vi "P2P SPI Slave.vi"   [LabVIEW 2015]
uses:
  <vilib>/Platform/TimedLoop/XDataNode/timing_clust.ctl
  <vilib>/Platform/TimedLoop/XDataNode/nitl_modes.ctl
  <vilib>/Platform/TimedLoop/XDataNode/wakeup.ctl
  <vilib>/rvi/Emulation/niFpgaSctlEmulationGetInTimedLoop.vi
  <vilib>/rvi/Emulation/niFpgaEmulationReportErrorSimple.vi
  <vilib>/rvi/Emulation/niFpgaGetClockAttributes.vi
  <vilib>/rvi/Emulation/niFpgaCriticalErrorInLSC.vi
  <vilib>/rvi/eio/common/nirviEmuTemplateMethod_errors.vi
  <vilib>/rvi/Emulation/niFpgaEmulationIsFPGAContextNoSignature.vi
  <vilib>/rvi/errors/niFpgaSetErrorForExecOnDevCompSimple.vi
  <vilib>/rvi/eio/common/nirviEmuReportErrorAndStop.vi
  <vilib>/rvi/DataTransferAndStorage/Container/Common/niFpgaContainerGetUniqueNameForEmu.vi
  <vilib>/rvi/FIFO/Fifo_Resource/nirvififoEmulationSetSize.vi
  <vilib>/rvi/FIFO/Fifo_Resource/nirviFifoEmulationQueueMgr.vi
  <instcachedir>/0/nirviFifoEmulationQueueMgr_E5CAEC123FF24DC58D834DCA3CDAA9B5.lvgen/nirviFifoEmulationQueueMgr_E5CAEC123FF24DC58D834DCA3CDAA9B5_001.vi
  <vilib>/rvi/FIFO/Fifo_Resource/nirvififoEmulationDetermineInputValidOut.vi
  <vilib>/rvi/FIFO/Fifo_Resource/nirvififoEmulationCreateLock.vi
  <vilib>/rvi/Emulation/niFpgaProcessEmulError.vi
  <vilib>/rvi/FIFO/Fifo_Resource/nirvififoEmulationObtainLock.vi
  <vilib>/rvi/FIFO/Fifo_Resource/nirvififoEmulationReleaseLock.vi
  <vilib>/rvi/occurrence/nirviWaitOnOccurrenceBase.vi
  <vilib>/rvi/errors/nirviReportUnexpectedCaseInternalError.vi
  <vilib>/rvi/errors/nirviReportUnexpectedCaseInternalError (U32).vi
  <vilib>/Platform/TimedLoop/XDataNode/XDataNode.xnode
  <vilib>/eio/EIONode/EIONode.xnode
  <vilib>/rvi/DataTransferAndStorage/Container/XNode/niFpgaContainer.xnode
  <vilib>/rvi/FIFO/Fifo_Resource/nirvififoEmulationWrite.vi
  <vilib>/Platform/TimedLoop/XDataNode/XDNodeRunTimeDep.lvlib
types:
  T1 = typedef "XDNodeRunTimeDep.lvlib/timing_clust.ctl" = cluster{"Expected End [f-1]":u64, "Actual End [f-1]":u64, "Finished Late? [f-1]":bool, "Expected End [i-1]":u64, "Actual End [i-1]":u64, "Finished Late? [i-1]":bool, "Expected Start [i]":u64, "Actual Start [i]":u64, "Expected Start [f]":u64, "Actual Start [f]":u64, "Source Name":string, "Structure Name":string, "Period":i64, "Deadline":i64, "Offset":i64, "Start":i64, "Priority":i32, "Timeout":i32, "Mode":T2, "Wakeup Reason":T3, "Error":errorcluster, "Source Type":string, "Secondary Source Type":string, "Global End Time":u64, "Global Start Time":u64, "Frame Duration":u64, "Iteration Duration":u64, "Assigned CPU":i32, "I/O Scan Engine Mode":u32}
  T2 = typedef "XDNodeRunTimeDep.lvlib/nitl_modes.ctl" = enum32{"No Change", "Process missed periods, maintain original phase", "Discard missed periods, maintain original phase", "Process missed periods, ignore original phase", "Discard missed periods, ignore original phase"}
  T3 = typedef "XDNodeRunTimeDep.lvlib/wakeup.ctl" = enum32{"Normal", "Aborted", "Asynchronous wakeup", "Timing source error", "Timed loop error", "Timeout"}
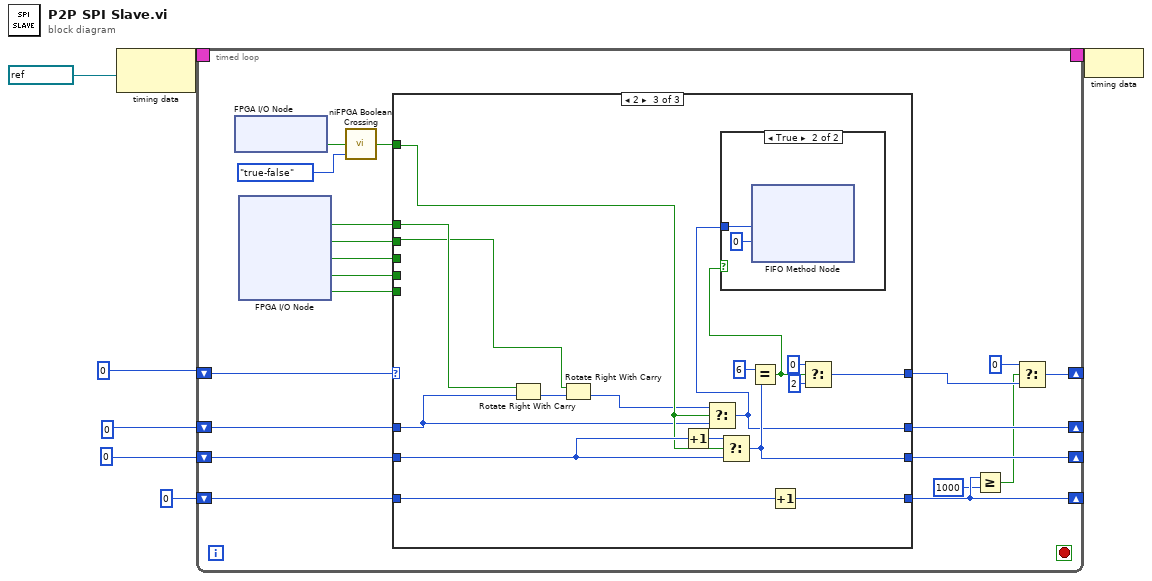
[diagram p0: block diagram]
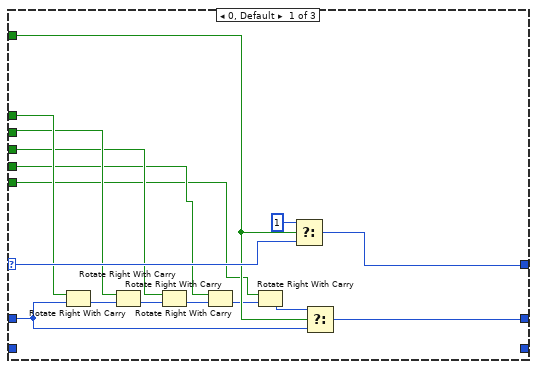
[diagram p2: hidden frame]
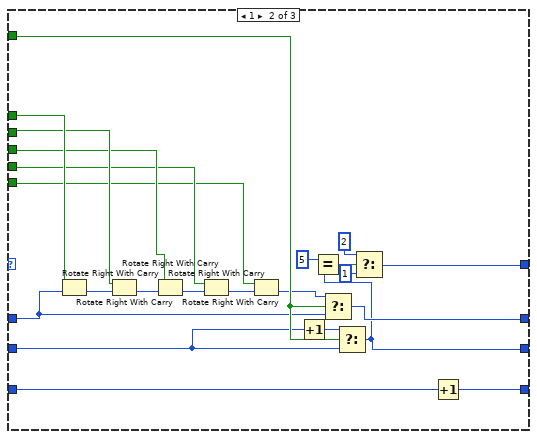
[diagram p3: hidden frame]
diagram:
  n1 = node-c288(refnum<k21> "80MHz" ("Source Name")) -> (w7:T1)
  n2 = timed-loop {
    timing: w7 -> [_]
    timing-out: [_] -> w6
    shift-right: [w9] -> _
    shift-left: u8 0 -> [w27]
    shift-right: [w21] -> _
    shift-left: u32 0 -> [w23]
    shift-right: [w11] -> _
    shift-left: u8 0 -> [w20]
    shift-right: [w14] -> _
    shift-left: 0 -> [w15]
    stop <- _ stop-if-true
    n3 = xnode "FPGA I/O Node"() -> ("PXI_Trig2"=w26:bool)  [unwired: 1 in, 1 out]
    n4 = xnode "FPGA I/O Node"() -> ("PXI_Trig3"=w22:bool, "PXI_Trig4"=w19:bool, "PXI_Trig5"=w18:bool, "PXI_Trig6"=w17:bool, "PXI_Trig7"=w16:bool)  [unwired: 5 in, 5 out]
    n5 = call <vilib>:"niFPGA Boolean Crossing.vi"("input"=w26, "direction"=enum8{"either", "false-true", "true-false"}."true-false") -> ("crossing"=w25:bool)  [unwired: 7 in]
    n6 = case shown="2" w27 {
      selector: w27 -> [w42 _ _]
      tunnel: w25 -> [w40 w65 w76]
      tunnel: [w43 w62 w81] -> w10
      tunnel: w23 -> [w33 w49 w70]
      tunnel: w22 -> [w32 w48 w69]
      tunnel: [w39 w64 w74] -> w21
      tunnel: w20 -> [_ w61 w80]
      tunnel: [_ w60 w79] -> w11
      tunnel: w19 -> [w31 w47 w68]
      tunnel: w18 -> [w30 w46 _]
      tunnel: w17 -> [w29 w45 _]
      tunnel: w16 -> [w28 w44 _]
      tunnel: [_ w55 w72] -> w14
      tunnel: w15 -> [_ w56 w73]
      frame 0, Default {
        n7 = Rotate Right With Carry(2:w33, 3:w32) -> (0:w35:u32)  [unwired: 1 out]
        n8 = Rotate Right With Carry(2:w35, 3:w31) -> (0:w36:u32)  [unwired: 1 out]
        n9 = Rotate Right With Carry(2:w36, 3:w30) -> (0:w37:u32)  [unwired: 1 out]
        n10 = Rotate Right With Carry(2:w37, 3:w29) -> (0:w38:u32)  [unwired: 1 out]
        n11 = Rotate Right With Carry(2:w38, 3:w28) -> (0:w34:u32)  [unwired: 1 out]
        n12 = Select(t=u8 1, s=w40, f=w42) -> (s? t:f=w43:u8)
        n13 = Select(t=w34, s=w40, f=w33) -> (s? t:f=w39:u32)
      }
      frame 1 {
        n14 = Rotate Right With Carry(2:w49, 3:w48) -> (0:w51:u32)  [unwired: 1 out]
        n15 = Rotate Right With Carry(2:w51, 3:w47) -> (0:w52:u32)  [unwired: 1 out]
        n16 = Rotate Right With Carry(2:w52, 3:w46) -> (0:w53:u32)  [unwired: 1 out]
        n17 = Rotate Right With Carry(2:w53, 3:w45) -> (0:w54:u32)  [unwired: 1 out]
        n18 = Rotate Right With Carry(2:w54, 3:w44) -> (0:w50:u32)  [unwired: 1 out]
        n19 = Increment(x=w61) -> (x+1=w66:u8)
        n20 = Select(t=w50, s=w65, f=w49) -> (s? t:f=w64:u32)
        n21 = Select(t=w66, s=w65, f=w61) -> (s? t:f=w60:u8)
        n22 = Equal?(x=u8 5, y=w60) -> (x = y?=w59:bool)
        n23 = Select(t=u8 2, s=w59, f=u8 1) -> (s? t:f=w62:u8)
        n24 = Increment(x=w56) -> (x+1=w55:i32)
      }
      frame 2 {
        n25 = Rotate Right With Carry(2:w70, 3:w69) -> (0:w71:u32)  [unwired: 1 out]
        n26 = Rotate Right With Carry(2:w71, 3:w68) -> (0:w67:u32)  [unwired: 1 out]
        n27 = Increment(x=w80) -> (x+1=w83:u8)
        n28 = Select(t=w67, s=w76, f=w70) -> (s? t:f=w74:u32)
        n29 = Select(t=w83, s=w76, f=w80) -> (s? t:f=w79:u8)
        n30 = Equal?(x=u8 6, y=w79) -> (x = y?=w75:bool)
        n31 = case shown="True" w75 {
          tunnel: w74 -> [_ w84]
          frame False {
          }
          frame True {
            n32 = xnode ("FIFO Method Node")("Element"=w84, "Timeout"=0) -> ()  [unwired: 1 in, 2 out]
          }
        }
        n33 = Increment(x=w73) -> (x+1=w72:i32)
        n34 = Select(t=u8 0, s=w75, f=u8 2) -> (s? t:f=w81:u8)
      }
    }
    n35 = Greater Or Equal?(x=w14, y=1000) -> (x >= y?=w8:bool)
    n36 = Select(t=u8 0, s=w8, f=w10) -> (s? t:f=w9:u8)
  }
  n37 = node-c288(w6) -> ()
